vi "LM Frequency Filter.vi"(6 "Observed LM Array":T1(array[cluster]), 8 "error in (no error)":errorcluster, 10 "SLAM In":T2) -> (0 "error out":errorcluster, 2 "SLAM Out":T2)   [LabVIEW 2009]
uses:
  Controls/SLAM.ctl
  <vilib>/Analysis/Matrix/Datatypes/RealMatrix.ctl
  <vilib>/Analysis/baseanly.llb/Real A x B.vi
  <vilib>/Analysis/Matrix/NI_Matrix.lvlib
  <vilib>/Analysis/NI_AALBase.lvlib
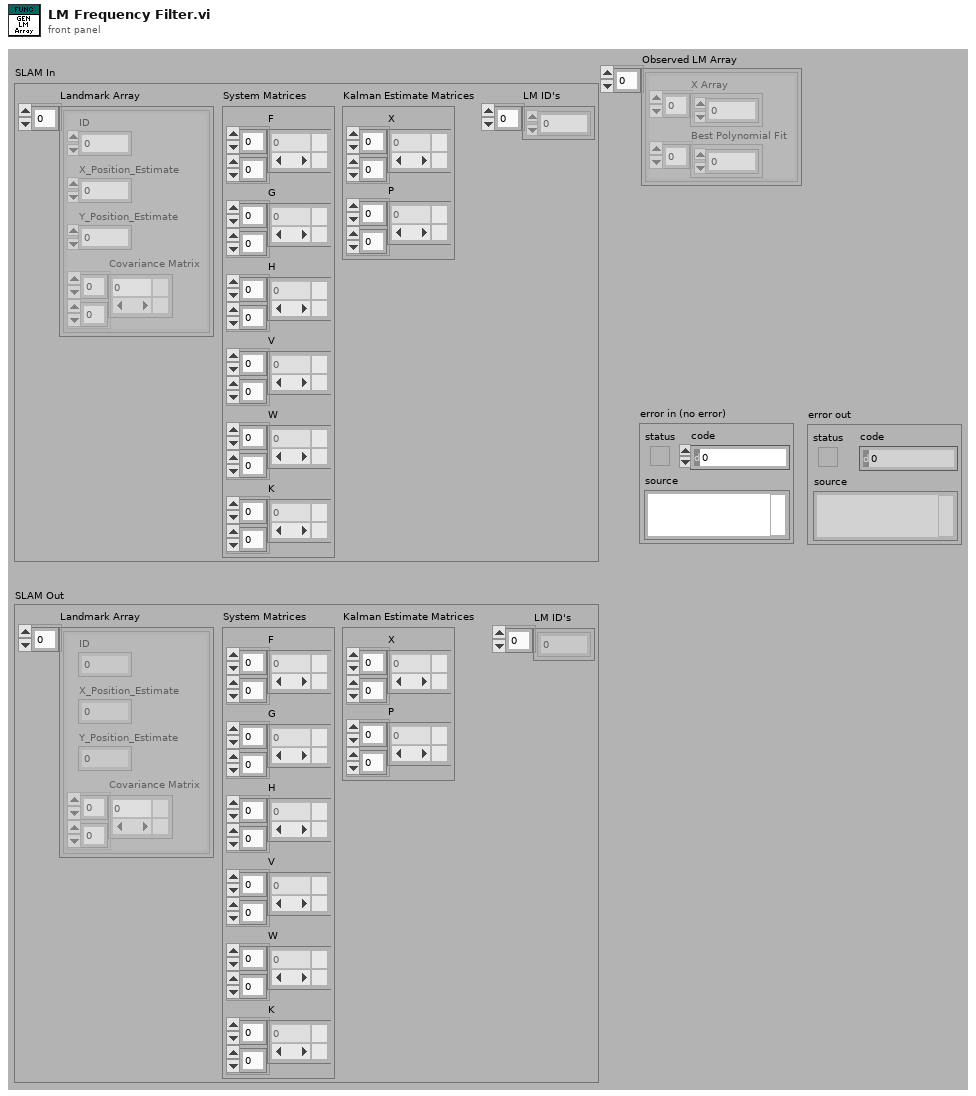
[diagram p1: front panel]
types:
  T1 = cluster{"X Array":dbl[], "Best Polynomial Fit":dbl[]}[]
  T2 = typedef "SLAM.ctl" = cluster{"Landmark Array":cluster{"ID":dbl, "X_Position_Estimate":dbl, "Y_Position_Estimate":dbl, "Covariance Matrix":T3}[], "System Matrices":cluster{"F":T3, "G":T3, "H":T3, "V":T3, "W":T3, "K":T3}, "Kalman Estimate Matrices":cluster{"X":T3, "P":T3}, "LM ID's":dbl[]}
  T3 = typedef "NI_Matrix.lvlib/RealMatrix.ctl" = dbl[][]
  T4 = cluster{"ID":dbl, "X_Position_Estimate":dbl, "Y_Position_Estimate":dbl, "Covariance Matrix":T3}[]
  T5 = cluster{"ID":dbl, "X_Position_Estimate":dbl, "Y_Position_Estimate":dbl, "Covariance Matrix":T3}
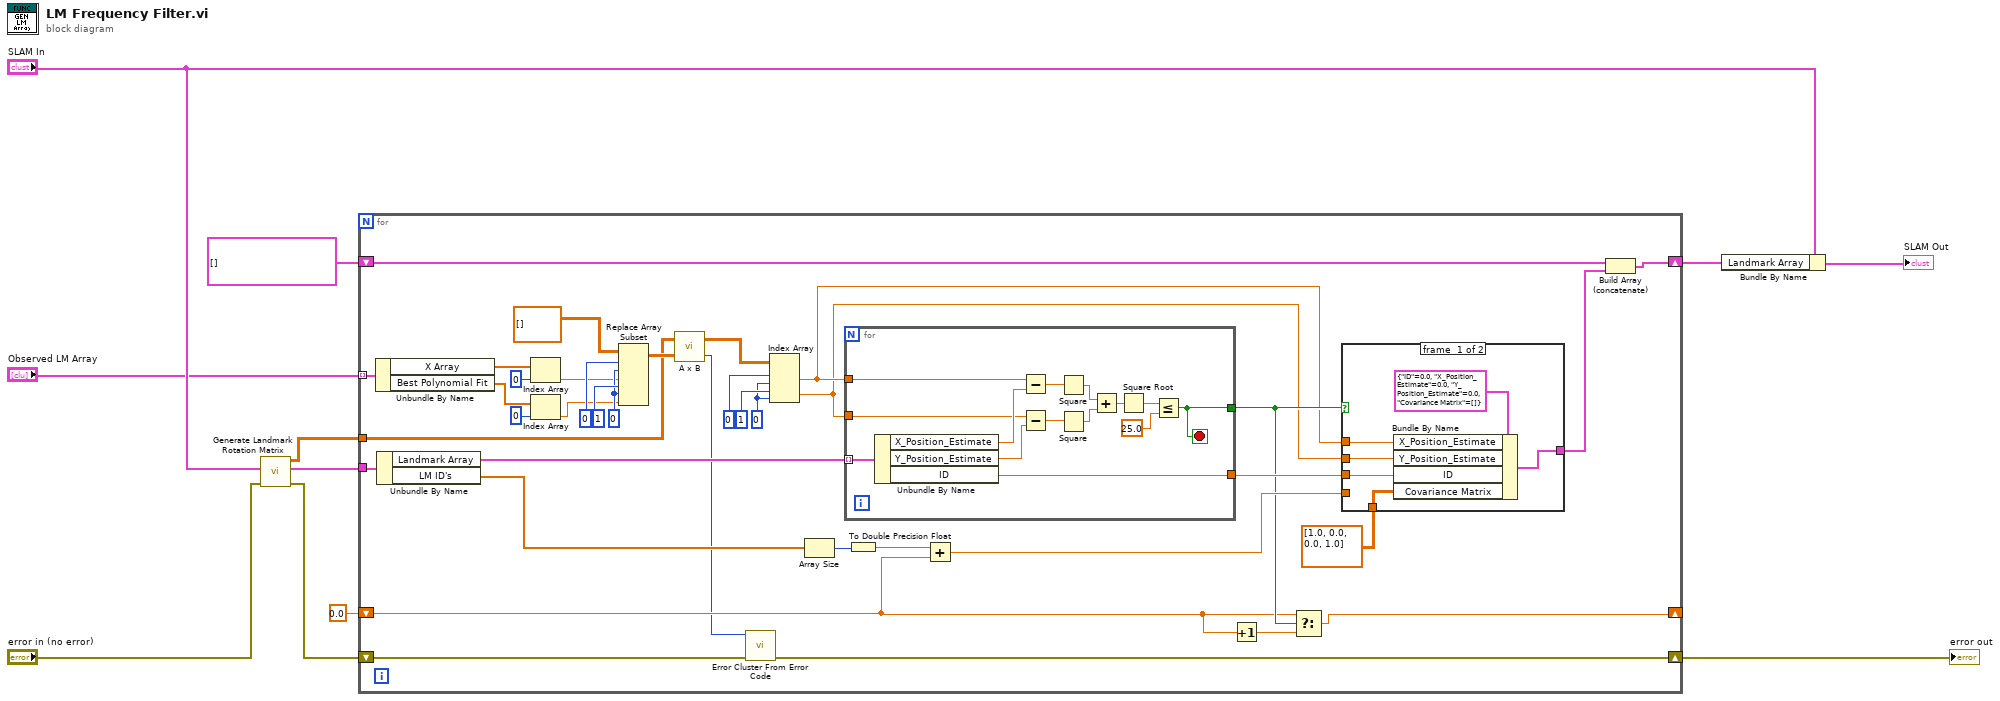
[diagram p0: block diagram]
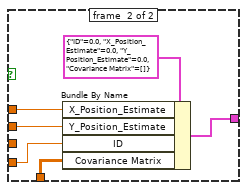
[diagram p2: hidden frame]
diagram:
  n1 = call "Generate Landmark Rotation Matrix.vi"("error in (no error)"="error in (no error)", "SLAM In"="SLAM In") -> ("error out"=w1:errorcluster, "SLAM Out"=w3:T2, "Rotation matrix"=w2:T3)  [unwired: 7 in]
  n2 = for {
    tunnel: "Observed LM Array" -> [w37] mode=indexing
    shift-right: [w46] -> w5
    shift-left: T4 [] ("appended array") -> [w48]
    tunnel: w3 -> [w44]
    shift-right: [w29] -> _
    shift-left: 0.0 ("double precision float") -> [w30]
    tunnel: w2 -> [w21]
    shift-right: [w14] -> w7
    shift-left: w1 -> [w15]
    w18 = 0 ("index (col)")
    w25 = 0 ("index (col)")
    n3 = Unbundle By Name(w37) -> ("X Array"=w40:dbl[], "Best Polynomial Fit"=w41:dbl[])
    n4 = Unbundle By Name(w44) -> ("Landmark Array"=w45:T4, "LM ID's"=w43:dbl[])
    n5 = Index Array(array=w40, index=0) -> (element=w23:dbl)
    n6 = Index Array(array=w41, index=0) -> (element=w22:dbl)
    n7 = Replace Array Subset(array=T3 [] ("matrix"), new element #1=w23, index (row) #1=0 ("index (col)"), index (col) #1=w25, new element #2=w22, index (row) #2=1 ("index (col)"), index (col) #2=w25) -> (w28:T3)
    n8 = call-poly <vilib>:"A x B.vi"("B"=w28, "A"=w21) -> ("error"=w16:i32, "A x B"=w17:T3)
    n9 = call <vilib>:"Error Cluster From Error Code.vi"("error in (no error)"=w15, "error code (0)"=w16) -> ("error out"=w14:errorcluster)  [unwired: 7 in]
    n10 = Index Array(array=w17, index (row) #1=0 ("index (col)"), index (col) #1=w18, index (row) #2=1 ("index (col)"), index (col) #2=w18) -> (element #1=w13:dbl, element #2=w12:dbl)
    n11 = Array Size(array=w43) -> (size(s)=w35:i32)
    n12 = for {
      tunnel: w45 -> [w74] mode=indexing
      tunnel: [w64] -> w32
      tunnel: [w63] -> w42
      tunnel: w13 -> [w62]
      tunnel: w12 -> [w61]
      stop <- w64 stop-if-true
      n13 = Unbundle By Name(w74) -> ("X_Position_Estimate"=w66:dbl, "Y_Position_Estimate"=w65:dbl, "ID"=w63:dbl)
      n14 = Subtract(x=w62, y=w66) -> (x-y=w72:dbl)
      n15 = Subtract(x=w61, y=w65) -> (x-y=w73:dbl)
      n16 = Square(x=w72) -> (x^2=w71:dbl)
      n17 = Square(x=w73) -> (x^2=w70:dbl)
      n18 = Add(x=w71, y=w70) -> (x+y=w69:dbl)
      n19 = Square Root(x=w69) -> (sqrt(x)=w68:dbl)
      n20 = Less Or Equal?(x=w68, y=25.0) -> (x <= y?=w64:bool)
    }
    n21 = To Double Precision Float(number=w35) -> (double precision float=w34:dbl)
    n22 = Add(x=w34, y=w30) -> (x+y=w33:dbl)
    n23 = Increment(x=w30) -> (x+1=w31:dbl)
    n24 = Select(t=w30, s=w32, f=w31) -> (s? t:f=w29:dbl)
    n25 = case shown="False" w32 {
      tunnel: [w53 w59] -> w47
      tunnel: w42 -> [w52 _]
      tunnel: T3 [[1.0, 0.0], [0.0, 1.0]] ("Covariance Matrix") -> [w51 w58]
      tunnel: w33 -> [_ w57]
      tunnel: w13 -> [w50 w56]
      tunnel: w12 -> [w49 w55]
      frame #0 {
        n26 = Bundle By Name(cluster=T5 {"ID"=0.0, "X_Position_Estimate"=0.0, "Y_Position_Estimate"=0.0, "Covariance Matrix"=[]} ("Landmarks"), "X_Position_Estimate"=w50, "Y_Position_Estimate"=w49, "ID"=w52, "Covariance Matrix"=w51) -> (w53:T5)
      }
      frame #1 {
        n27 = Bundle By Name(cluster=T5 {"ID"=0.0, "X_Position_Estimate"=0.0, "Y_Position_Estimate"=0.0, "Covariance Matrix"=[]} ("Landmarks"), "X_Position_Estimate"=w56, "Y_Position_Estimate"=w55, "ID"=w57, "Covariance Matrix"=w58) -> (w59:T5)
      }
    }
    n28 = Build Array (concatenate)(w48, w47) -> (w46:T4)
  }
  "error out" <- w7
  n29 = Bundle By Name(cluster="SLAM In", "Landmark Array"=w5) -> (→"SLAM Out":T2)
